vi "Read Loop Async.vi"(11 "Websocket Client in":refnum<class "Websocket Client.lvclass">) -> ()   [LabVIEW 2020]
uses:
  Websocket Client.lvclass/Websocket Client.ctl
  Websocket Client.lvclass
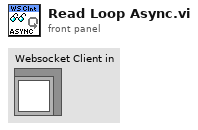
[diagram p1: front panel]
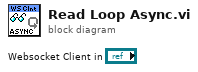
[diagram p0: block diagram]
diagram:
